vi "GetIntValue.vi"(2 "error in (no error)":errorcluster, 3 "Feature Name":string, 4 "IGXDevice":refnum<k24>) -> (0 "error out":errorcluster, 1 "Int Value":i32)   [LabVIEW 2013, in "GxLVlib.lvlib"]
uses:
  GxLVlib.lvlib
  F:/GxILibrary/Labview/trunk/private/dev/src/C#/x64/GxLVLib/dll/GxIAPINET.dll
  private/dev/src/C#/x64/GxLVLib/dll/GxIAPINET.dll
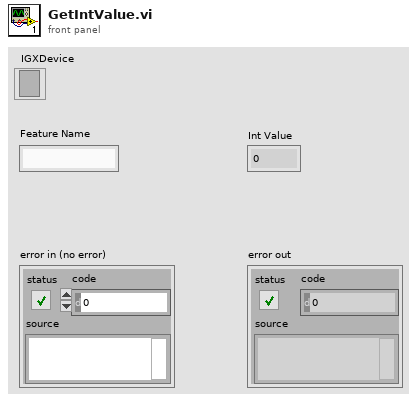
[diagram p1: front panel]
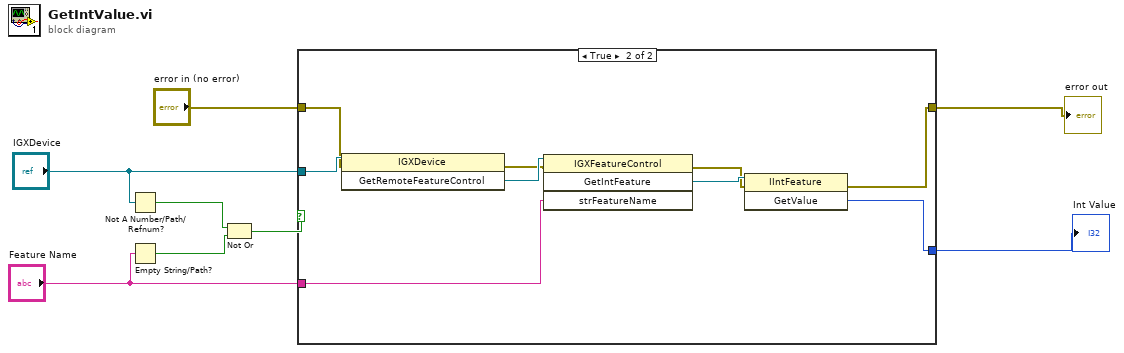
[diagram p0: block diagram]
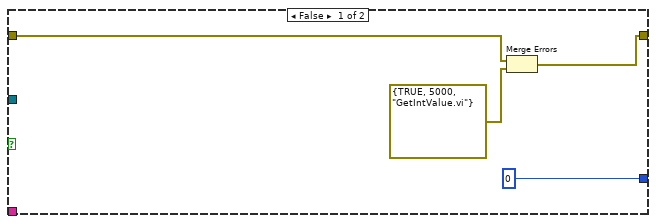
[diagram p2: hidden frame]
diagram:
  n1 = Not A Number/Path/Refnum?(number/path/refnum="IGXDevice") -> (NaN/Path/Refnum?=w8:bool)
  n2 = Empty String/Path?(string/path="Feature Name") -> (empty?=w7:bool)
  n3 = Not Or(1:w7, 2:w8) -> (0:w6:bool)
  n4 = case shown="True" w6 {
    tunnel: "error in (no error)" -> [w10 w16]
    tunnel: [w9 w13] -> w4
    tunnel: [0 w17] -> w3
    tunnel: "IGXDevice" -> [_ w21]
    tunnel: "Feature Name" -> [_ w19]
    frame False {
      n5 = Merge Errors(w10, errorcluster {TRUE, 5000, "GetIntValue.vi"}) -> (w9:errorcluster)
    }
    frame True {
      n6 = invoke class="IGXDevice" method="GetRemoteFeatureControl"(reference=w21, error in=w16) -> (error out=w15:errorcluster, "GetRemoteFeatureControl"=w20:refnum<k24>)  [unwired: 1 in, 1 out]
      n7 = invoke class="IGXFeatureControl" method="GetIntFeature"(reference=w20, error in=w15, "strFeatureName"=w19) -> (error out=w14:errorcluster, "GetIntFeature"=w18:refnum<k24>)  [unwired: 1 in, 2 out]
      n8 = invoke class="IIntFeature" method="GetValue"(reference=w18, error in=w14) -> (error out=w13:errorcluster, "GetValue"=w17:i64)  [unwired: 1 in, 1 out]
    }
  }
  "Int Value" <- w3
  "error out" <- w4
